vi "CBR_Player.vi"() -> ()   [LabVIEW 2012]
panel:
  out "text":string
  in  "VIA":path=path "/Kim/Users/crogers/Documents/LabVIEW Data/LVVIAGenerated/Demo1.vi  2013-12-18 14-09-36.via"
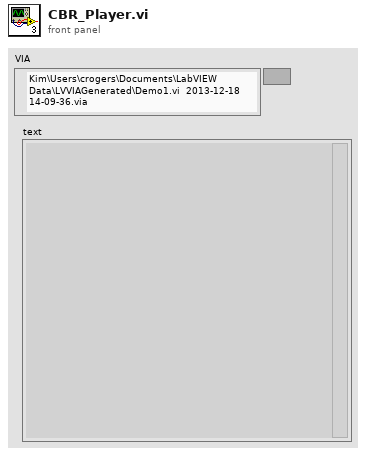
[diagram p1: front panel]
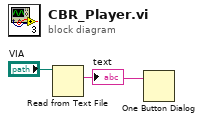
[diagram p0: block diagram]
diagram:
  n1 = Read from Text File(file (use dialog)="VIA") -> (text=w1:string)  [unwired: 3 in, 3 out]
  "text" <- w1
  n2 = One Button Dialog(message=w1) -> ()  [unwired: 1 in, 1 out]
